vi "Set MCS Index.vi"(8 "error in (no error)":errorcluster, 10 "MCS Index":i32, 11 "niDTS WLAN Dut Data in":refnum<class "niDTS WLAN Dut Data.lvclass">) -> (0 "error out":errorcluster, 3 "niDTS WLAN Dut Data out":refnum<class "niDTS WLAN Dut Data.lvclass">)   [LabVIEW 2015, in "niDTS WLAN.lvlib" / "niDTS WLAN Dut Data.lvclass"]
uses:
  niDTS WLAN Dut Data.lvclass
  niDTS WLAN Dut Data.lvclass/niDTS WLAN Dut Data.ctl
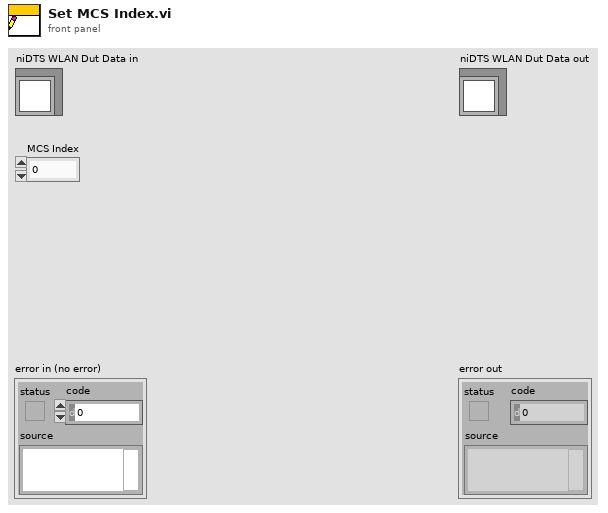
[diagram p1: front panel]
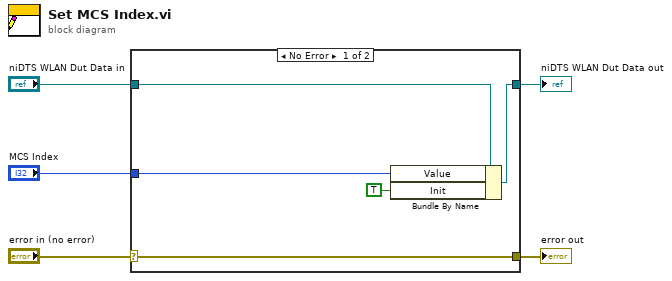
[diagram p0: block diagram]
diagram:
  n1 = case shown="No Error" "error in (no error)" {
    selector: "error in (no error)" -> [w10 w11]
    tunnel: [w10 w11] -> w4
    tunnel: [w8 w12] -> w2
    tunnel: "niDTS WLAN Dut Data in" -> [w9 w12]
    tunnel: "MCS Index" -> [w7 _]
    frame No Error {
      n2 = Bundle By Name(cluster=w9, "Value"=w7, "Init"=TRUE ("MCS Index.Init")) -> (w8:refnum<class "niDTS WLAN Dut Data.lvclass">)
    }
    frame Error {
    }
  }
  "error out" <- w4
  "niDTS WLAN Dut Data out" <- w2
